vi "SetVISAResourceName.vi"(8 "error in (no error)":errorcluster, 10 "VISA resource name":refnum<visa-resource-name>, 11 "object in":refnum<class "PowerSupply.lvclass">) -> (0 "error out":errorcluster, 3 "object out":refnum<class "PowerSupply.lvclass">)   [LabVIEW 2023, in "HardwareAbstractionLayer_LVOOP.lvlib" / "PowerSupply.lvclass"]
uses:
  PowerSupply.lvclass
  PowerSupply.lvclass/PowerSupply.ctl
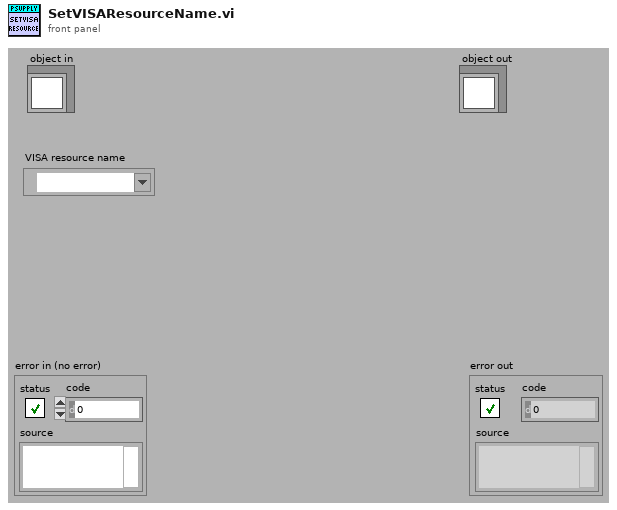
[diagram p1: front panel]
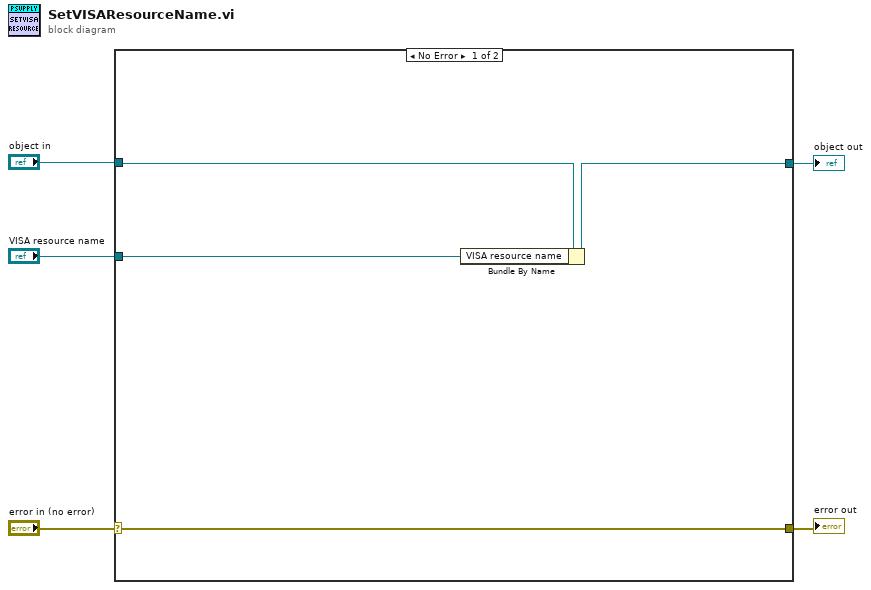
[diagram p0: block diagram]
diagram:
  n1 = case shown="No Error" "error in (no error)" {
    selector: "error in (no error)" -> [w8 w11]
    tunnel: [w8 w11] -> w4
    tunnel: [w6 w10] -> w2
    tunnel: "object in" -> [w7 w10]
    tunnel: "VISA resource name" -> [w9 _]
    frame No Error {
      n2 = Bundle By Name(cluster=w7, "VISA resource name"=w9) -> (w6:refnum<class "PowerSupply.lvclass">)
    }
    frame Error {
    }
  }
  "error out" <- w4
  "object out" <- w2
